vi "Read Exist Status.vi"(5 "Username":string, 6 "Password":string, 7 "Address":string, 8 "Error In":errorcluster) -> (0 "Error Out":errorcluster)   [LabVIEW 2018, in "Tests.lvlib" / "Channel.lvlib"]
uses:
  Channel.lvlib
  src/Toolkit/API/Channel/Channel.lvclass/Channel.ctl
  src/Toolkit/API/Session/Session.lvclass/Session.ctl
  src/Toolkit/API/SSH/SSH.lvclass/SSH.ctl
  src/Toolkit/API/Session/Utility/Read Shared Library.vi
  src/Toolkit/API/SSH/Utility/Read Shared Library.vi
  <vilib>/addons/_JKI Toolkits/Caraya/classes/Test/Test.lvclass
  <vilib>/addons/_JKI Toolkits/Caraya/classes/Assert/Assert.lvclass
  src/Toolkit/API/Channel/Channel.lvclass
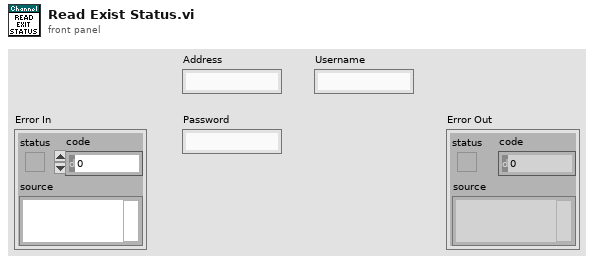
[diagram p1: front panel]
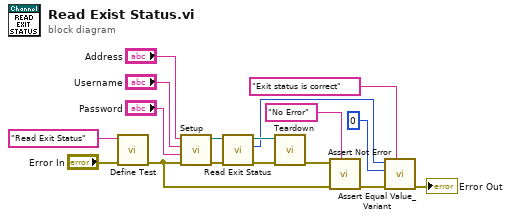
[diagram p0: block diagram]
diagram:
  n1 = call <vilib>:"Define Test.vi"("error in (no error)"="Error In", "Label (VI Title)"="Read Exit Status") -> ("error out"=w14:errorcluster)  [unwired: 9 in]
  n2 = call "Setup.vi"("Error In"=w14, "Password"="Password", "Username"="Username", "Address"="Address") -> ("Error Out"=w6:errorcluster, "Channel"=w9:refnum<class "Channel.lvclass">)  [unwired: 6 in]
  n3 = call "Read Exit Status.vi"("Error In"=w6, "Channel In"=w9) -> ("Error Out"=w7:errorcluster, "Exit Status"=w2:i32, "Channel Out"=w8:refnum<class "Channel.lvclass">)  [unwired: 7 in]
  n4 = call "Teardown.vi"("Error In"=w7, "Channel"=w8) -> ("Error Out"=w10:errorcluster)  [unwired: 9 in]
  n5 = call <vilib>:"Assert Not Error.vi"("Label"="No Error", "error in (no error)"=w14, "Not Error?"=w10) -> ("error out"=w5:errorcluster)  [unwired: 8 in]
  n6 = call <vilib>:"Assert Equal Value_Variant.vi"("Label"="Exit status is correct", "error in (no error)"=w5, "Y"=0 ("Exit Status"), "X"=w2) -> ("error out"=→"Error Out":errorcluster)  [unwired: 7 in]
